vi "CN0tot.vi"(1 "C/N0d (dBHz)":dbl, 2 "C/N0u (dBHz)":dbl) -> (0 "C/N0tot (dBHz)":dbl)   [LabVIEW 2015]
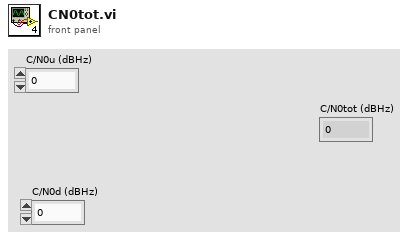
[diagram p1: front panel]
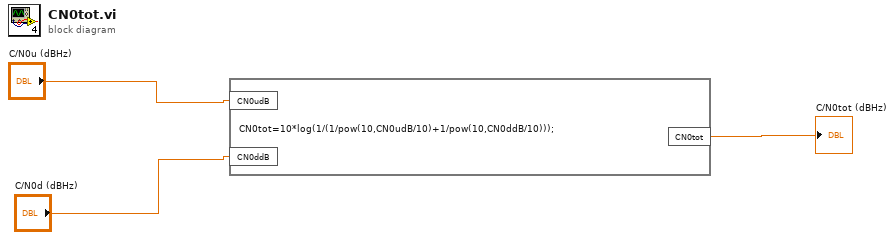
[diagram p0: block diagram]
diagram:
  n1 = formula code="CN0tot=10*log(1/(1/pow(10,CN0udB/10)+1/pow(10,CN0ddB/10)));"("CN0udB"="C/N0u (dBHz)", "CN0ddB"="C/N0d (dBHz)") -> ("CN0tot"=→"C/N0tot (dBHz)":dbl)
